vi "listen.vi"(8 "error in (no error)":errorcluster, 11 "tcp socket fd":i32) -> (0 "error out":errorcluster, 3 "success":u16)   [LabVIEW 2015]
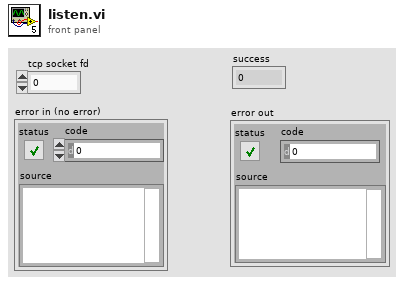
[diagram p1: front panel]
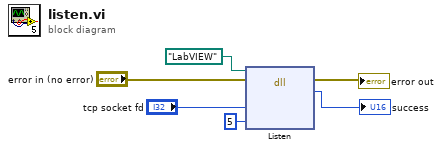
[diagram p0: block diagram]
diagram:
  n1 = dll-call lib="LabVIEW" fn="Listen"(path in=path "LabVIEW", error in="error in (no error)", "sockfd"="tcp socket fd", "backlog"=u16 5) -> (error out=→"error out":errorcluster, "success"=→"success":u16)  [unwired: 3 in, 1 out]
